vi "Ad模拟.vi"(1 "Ad通道号":u8=1 min=1 max=8) -> (0 "仿真值":dbl format="%#_7g")   [LabVIEW 2010]
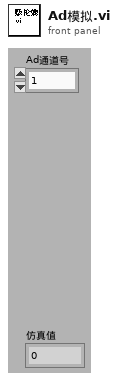
[diagram p1: front panel]
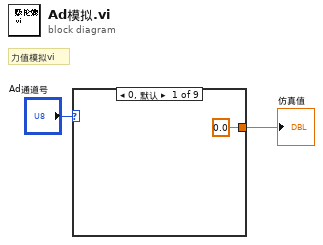
[diagram p0: block diagram]
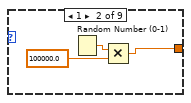
[diagram p2: hidden frame]
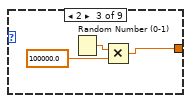
[diagram p3: hidden frame]
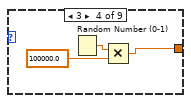
[diagram p4: hidden frame]
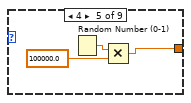
[diagram p5: hidden frame]
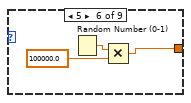
[diagram p6: hidden frame]
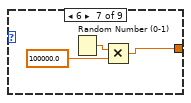
[diagram p7: hidden frame]
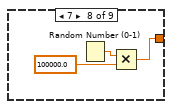
[diagram p8: hidden frame]
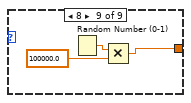
[diagram p9: hidden frame]
diagram:
  # "力值模拟vi"
  n1 = case shown="0, 默认" "Ad通道号" {
    tunnel: [0.0 w4 w7 w10 w13 w16 w19 w22 w25] -> w1
    frame 0, Default {
    }
    frame 1 {
      n2 = Random Number (0-1)() -> (number: 0 to 1=w6:dbl)
      n3 = Multiply(x=w6, y=100000.0) -> (x*y=w4:dbl)
    }
    frame 2 {
      n4 = Random Number (0-1)() -> (number: 0 to 1=w9:dbl)
      n5 = Multiply(x=w9, y=100000.0) -> (x*y=w7:dbl)
    }
    frame 3 {
      n6 = Random Number (0-1)() -> (number: 0 to 1=w12:dbl)
      n7 = Multiply(x=w12, y=100000.0) -> (x*y=w10:dbl)
    }
    frame 4 {
      n8 = Random Number (0-1)() -> (number: 0 to 1=w15:dbl)
      n9 = Multiply(x=w15, y=100000.0) -> (x*y=w13:dbl)
    }
    frame 5 {
      n10 = Random Number (0-1)() -> (number: 0 to 1=w18:dbl)
      n11 = Multiply(x=w18, y=100000.0) -> (x*y=w16:dbl)
    }
    frame 6 {
      n12 = Random Number (0-1)() -> (number: 0 to 1=w21:dbl)
      n13 = Multiply(x=w21, y=100000.0) -> (x*y=w19:dbl)
    }
    frame 7 {
      n14 = Random Number (0-1)() -> (number: 0 to 1=w24:dbl)
      n15 = Multiply(x=w24, y=100000.0) -> (x*y=w22:dbl)
    }
    frame 8 {
      n16 = Random Number (0-1)() -> (number: 0 to 1=w27:dbl)
      n17 = Multiply(x=w27, y=100000.0) -> (x*y=w25:dbl)
    }
  }
  "仿真值" <- w1
